vi "HH_3axis_SimpleMotion.vi"() -> ()   [LabVIEW 2016]
uses:
  Motion/EnableMultiple.vi
  Motion/MoveIncMultiple.vi
  Motion/WaitMultiple.vi
  Motion/DisableMultiple.vi
panel:
  out "Position 3":string
  in  "Distance 3":dbl=25.0
  in  "Speed 3":dbl=5.0
  in  "Axis Name 3":string="Z"
  out "Position 2":string
  in  "Distance 2":dbl=100.0
  in  "Speed 2":dbl=12.5
  in  "Axis Name 2":string="Y"
  out "Position":string
  in  "Distance":dbl=150.0
  in  "Speed":dbl=25.0
  in  "Axis Name":string="X"
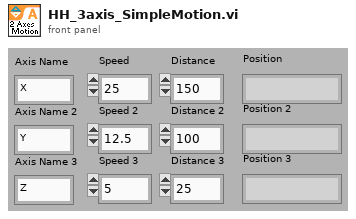
[diagram p1: front panel]
types:
  T1 = typedef "ControllerDiagPacket.ctl" = cluster{"Number of Diag Packets":i32, "Axes":T2[], "error":errorcluster}
  T2 = typedef "AxisDiagPacket.ctl" = cluster{"Axis Name":string, "Analog Input 0":dbl, "Analog Input 1":dbl, "Axis Fault (num)":i32, "Axis Fault (str)":string, "Axis Fault (bits)":cluster{"AmplifierFault":bool, "AmplifierTemperatureFault":bool, "CcwEndOfTravelLimitFault":bool, "CcwSoftwareLimitFault":bool, "CommunicationLostFault":bool, "CwEndOfTravelLimitFault":bool, "CwSoftwareLimitFault":bool, "EmergencyStopFault":bool, "EncoderFault":bool, "ExternalFault":bool, "FeedbackScalingFault":bool, "GantryMisalignFault ":bool, "HallSensorFault":bool, "InPositionTimeoutFault":bool, "MarkerSearchFault":bool, "MaxVelocityCommandFault":bool, "MissedInterruptFault":bool, "MotorTemperatureFault":bool, "None":bool, "OverCurrentFault":bool, "PositionErrorFault":bool, "PositionFeedbackFault":bool, "PowerSupplyFault":bool, "ProbeInputFault":bool, "SafeZoneFault":bool, "VelocityErrorFault":bool, "VelocityFeedbackFault":bool, "VoltageClampFault":bool}, "Axis Status (num)":i32, "Axis Status (str)":string, "Axis Status (bits)":cluster{"BacklashActive":bool, "CalibrationEnabled1D":bool, "CalibrationEnabled2D":bool, "CommandValid":bool, "DriveAbortPending":bool, "DrivePending":bool, "Enabling":bool, "GainMappingEnabled":bool, "GantryAligned":bool, "GantryRealigning":bool, "Homed":bool, "Homing":bool, "IFOVEnabled":bool, "JogGenerating":bool, "Jogging":bool, "JoystickControl":bool, "MasterSlaveControl":bool, "MotionBlocked":bool, "MotionClamped":bool, "MoveDone":bool, "None":bool, "NotVirtual":bool, "Profiling":bool, "Stability0":bool, "Stability1":bool, "TrajectoryFiltering":bool, "WaitDone":bool}, "Current Command":sgl, "Current Error":sgl, "Current Feedback":sgl, "Digital Inputs":i32, "Digital Outputs":i32, "Drive Status":i32, "Drive Status (str)":string, "Drive Status (bits)":cluster{"AccelerationPhase":bool, "AutofocusActive":bool, "BrakeOutput":bool, "CcwEndOfTravelLimitInput":bool, "CosineEncoderError":bool, "CurrentClamp":bool, "CwEndOfTravelLimitInput":bool, "DecelerationPhase":bool, "DualLoopActive":bool, "EmergencyStopInput":bool, "Enabled":bool, "EncoderClipping":bool, "GalvoCalibrationEnabled":bool, "GalvoPowerCorrection":bool, "HallAInput":bool, "HallBInput":bool, "HallCInput":bool, "HighResolutionMode":bool, "HomeLimitInput":bool, "InPosition":bool, "InPosition2":bool, "MarkerInput":bool, "MarkerLatch":bool, "MoveActive":bool, "NoMotorSupply":bool, "None":bool, "PowerLimiting":bool, "ProgrammingFlash":bool, "ProgrammingMXH":bool, "PSOHaltLatch":bool, "ServoControl":bool, "SineEncoderError":bool}, "Position Feedback Auxiliary":dbl, "Position Command":dbl, "Position Error":dbl, "Position Feedback":dbl, "Program Position Command":dbl, "Program Position Error":dbl, "Program Position Feedback":dbl, "Velocity Command":dbl, "Velocity Error":dbl, "Velocity Feedback":dbl}
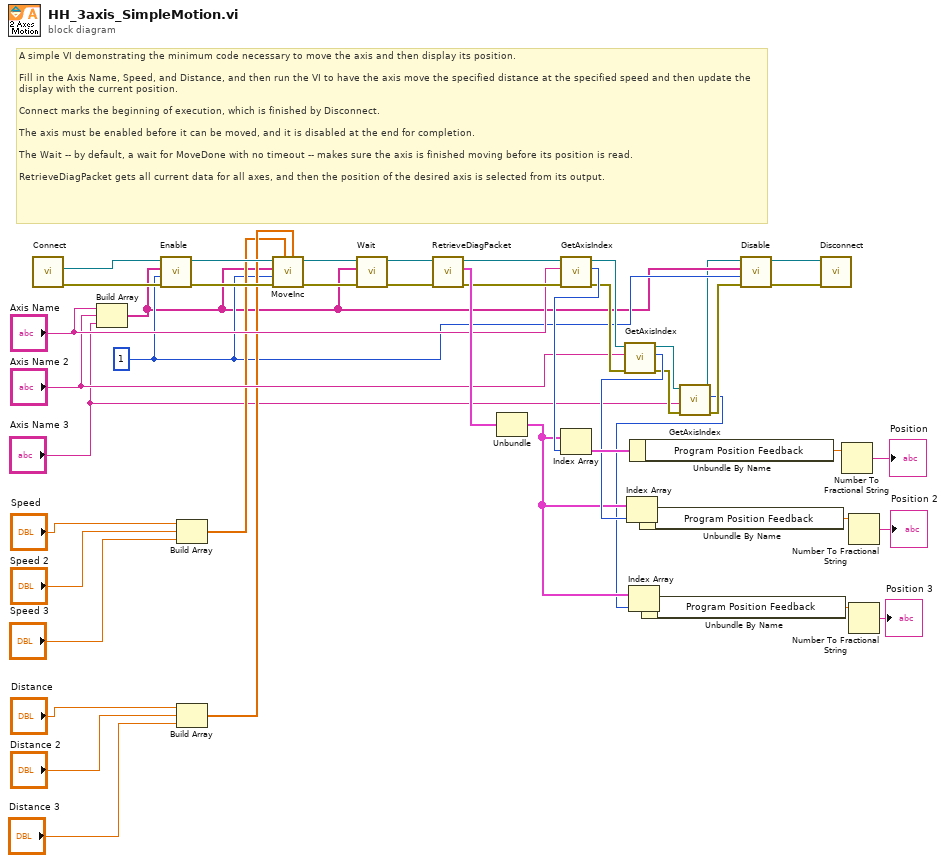
[diagram p0: block diagram]
diagram:
  w18 = 1 ("taskNumber")
  # "A simple VI demonstrating the minimum code necessary to move the axis and then display its position.\n\nFill in the Axis Name, Speed, and Distance, and then run the VI to have the axis move the specified distance at the specified speed and then update the display with the current position.\n\nConnect marks the beginning of execution, which is finished by Disconnect.\n\nThe axis must be enabled before it can be moved, and it is disabled at the end for completion.\n\nThe Wait -- by default, a wait for MoveDone with no timeout -- makes sure the axis is finished moving before its position is read.\n\nRetrieveDiagPacket gets all current data for all axes, and then the position of the desired axis is selected from its output."
  n1 = call "Connect.vi"() -> ("error out"=w26:errorcluster, "controller"=w27:refnum<k24>)  [unwired: 10 in]
  n2 = Build Array("Axis Name", "Axis Name 2", "Axis Name 3") -> (w13:string[])
  n3 = call-poly "Enable.vi"("error in (no error)"=w26, "taskId"=w18, "axis names"=w13, "controller in"=w27) -> ("error out"=w25:errorcluster, "controller out"=w24:refnum<k24>)  [unwired: 6 in]
  n4 = Build Array("Speed", "Speed 2", "Speed 3") -> (w19:dbl[])
  n5 = Build Array("Distance", "Distance 2", "Distance 3") -> (w20:dbl[])
  n6 = call-poly "MoveInc.vi"("distances"=w20, "speeds"=w19, "error in (no error)"=w25, "taskId"=w18, "axis names"=w13, "controller in"=w24) -> ("error out"=w17:errorcluster, "controller out"=w15:refnum<k24>)  [unwired: 4 in]
  n7 = call-poly "Wait.vi"("error in (no error)"=w17, "axis names"=w13, "controller in"=w15) -> ("error out"=w16:errorcluster, "controller out"=w14:refnum<k24>)  [unwired: 6 in, 1 out]
  n8 = call "RetrieveDiagPacket.vi"("error in (no error)"=w16, "Controller In"=w14) -> ("error out"=w43:errorcluster, "ControllerDiagPacket"=w45:T1, "Controller Out"=w34:refnum<k24>)  [unwired: 7 in]
  n9 = Unbundle(w45) -> ("Axes"=w9:T2[])  [unwired: 2 out]
  n10 = call "GetAxisIndex.vi"("error in (no error)"=w43, "axis name"="Axis Name", "controller in"=w34) -> ("error out"=w35:errorcluster, "axis index"=w42:i32, "controller out"=w22:refnum<k24>)  [unwired: 6 in]
  n11 = Index Array(array=w9, index=w42) -> (element=w41:T2)
  n12 = call "GetAxisIndex.vi"("error in (no error)"=w35, "axis name"="Axis Name 2", "controller in"=w22) -> ("error out"=w8:errorcluster, "axis index"=w36:i32, "controller out"=w5:refnum<k24>)  [unwired: 6 in]
  n13 = Index Array(array=w9, index=w36) -> (element=w37:T2)
  n14 = Unbundle By Name(w41) -> ("Program Position Feedback"=w40:dbl)
  n15 = Unbundle By Name(w37) -> ("Program Position Feedback"=w39:dbl)
  n16 = call "GetAxisIndex.vi"("error in (no error)"=w8, "axis name"="Axis Name 3", "controller in"=w5) -> ("error out"=w7:errorcluster, "axis index"=w6:i32, "controller out"=w4:refnum<k24>)  [unwired: 6 in]
  n17 = Index Array(array=w9, index=w6) -> (element=w12:T2)
  n18 = Unbundle By Name(w12) -> ("Program Position Feedback"=w11:dbl)
  n19 = call-poly "Disable.vi"("error in (no error)"=w7, "taskId"=w18, "axis names"=w13, "controller in"=w4) -> ("error out"=w23:errorcluster, "controller out"=w21:refnum<k24>)  [unwired: 6 in]
  n20 = call "Disconnect.vi"("error in (no error)"=w23, "controller"=w21) -> ()  [unwired: 9 in, 1 out]
  n21 = Number To Fractional String(number=w40) -> (F-format string=→"Position":string)  [unwired: 3 in]
  n22 = Number To Fractional String(number=w39) -> (F-format string=→"Position 2":string)  [unwired: 3 in]
  n23 = Number To Fractional String(number=w11) -> (F-format string=→"Position 3":string)  [unwired: 3 in]
